vi "SwapInstanceVIUnusedName2 59.vi"(6 "Bindata & descr in":T1, 7 "type":dbl, 8 "error in (no error)":errorcluster, 9 "dims":u8=3 min=1 max=3, 11 "kwarg_name":string="testarg") -> (0 "error out":errorcluster, 1 "Array 3D":dbl[][][](array[numeric]) format="%.2f", 2 "Array 2D":dbl[][](array[numeric]) format="%.2f", 3 "Array 1D":dbl[](array[numeric]) format="%.2f", 4 "Bindata & descr out":T1, 5 "bindata":u8[](array[numeric]))   [LabVIEW 2018]
uses:
  Bindata&description.ctl
  Bindata description.ctl
  bd6e6838-feb3-450b-96c3-bd7f3c631cc0.vi
  c6590a7f-93ce-4676-a9a0-c02eb749ea57.vi
  2ac210e2-aaf9-4bd7-a45e-3c20e6b86e14.vi
  031c4b19-b0b4-4976-a006-513195ae331f.vi
  c6590a7f-93ce-4676-a9a0-c02eb749ea57.vi/81d0cee2-99a7-4483-80a4-f543021384a2.vi
  2ac210e2-aaf9-4bd7-a45e-3c20e6b86e14.vi/3e6cde74-74c6-4a84-975f-0badd6472140.vi
  031c4b19-b0b4-4976-a006-513195ae331f.vi/10b3e457-c1b7-418a-95f2-1100ecc8746c.vi
  c6590a7f-93ce-4676-a9a0-c02eb749ea57.vi/81d0cee2-99a7-4483-80a4-f543021384a2.vi/ea25def5-b33f-46c8-9800-af2b1901f06e.vi
  2ac210e2-aaf9-4bd7-a45e-3c20e6b86e14.vi/3e6cde74-74c6-4a84-975f-0badd6472140.vi/823fcfe4-69d6-4cbf-9d8a-245ae98e7b4b.vi
  031c4b19-b0b4-4976-a006-513195ae331f.vi/10b3e457-c1b7-418a-95f2-1100ecc8746c.vi/6efc0fc5-4d4d-4c58-9f04-a5d9debc7065.vi
  c6590a7f-93ce-4676-a9a0-c02eb749ea57.vi/81d0cee2-99a7-4483-80a4-f543021384a2.vi/ea25def5-b33f-46c8-9800-af2b1901f06e.vi/f81dd119-ed08-4cbe-a226-a8bb7977346c.vi
  2ac210e2-aaf9-4bd7-a45e-3c20e6b86e14.vi/3e6cde74-74c6-4a84-975f-0badd6472140.vi/823fcfe4-69d6-4cbf-9d8a-245ae98e7b4b.vi/7a113b46-2298-43de-997a-f25a7eda3428.vi
  031c4b19-b0b4-4976-a006-513195ae331f.vi/10b3e457-c1b7-418a-95f2-1100ecc8746c.vi/6efc0fc5-4d4d-4c58-9f04-a5d9debc7065.vi/cf528bb0-7ade-42af-b83d-2163692bdb4a.vi
  check ID validity.vi
  LV-Julia_ZMQ-Roundtrip_lib.lvlib
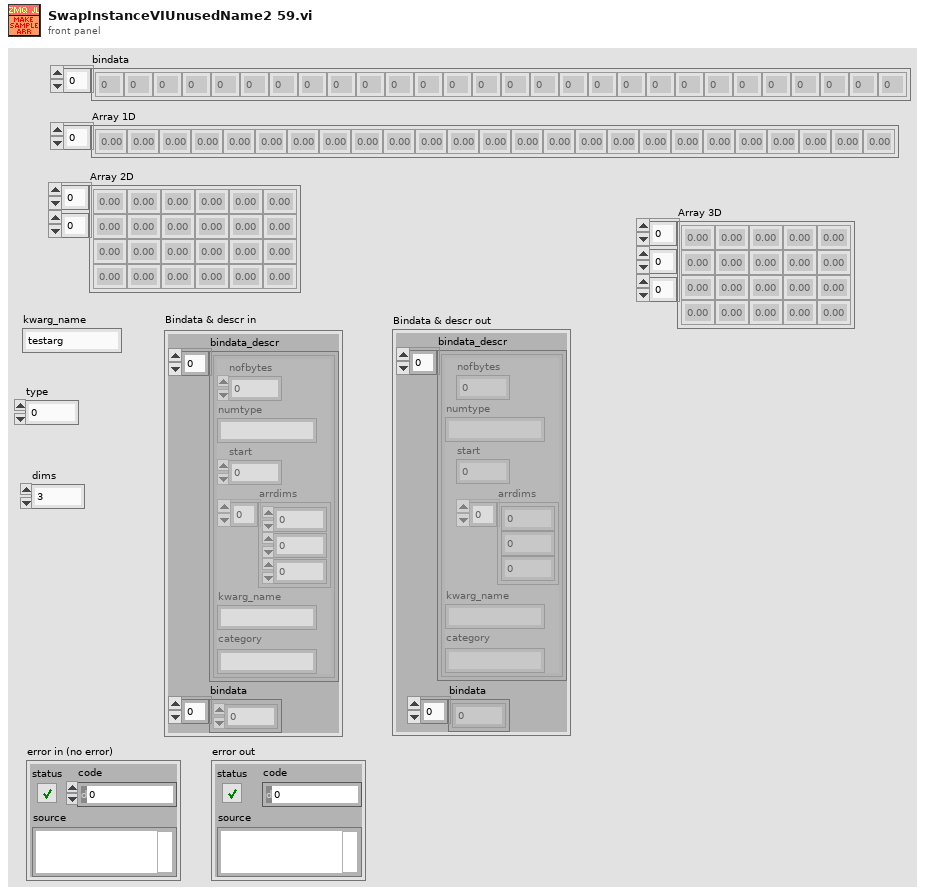
[diagram p1: front panel]
types:
  T1 = typedef "Bindata&description.ctl" = cluster{"bindata_descr":T2[], "bindata":u8[]}
  T2 = typedef "LV-Julia_ZMQ-Roundtrip_lib.lvlib/Bindata description.ctl" = cluster{"nofbytes":i32, "numtype":string, "start":i32, "arrdims":i32[], "kwarg_name":string, "category":string}
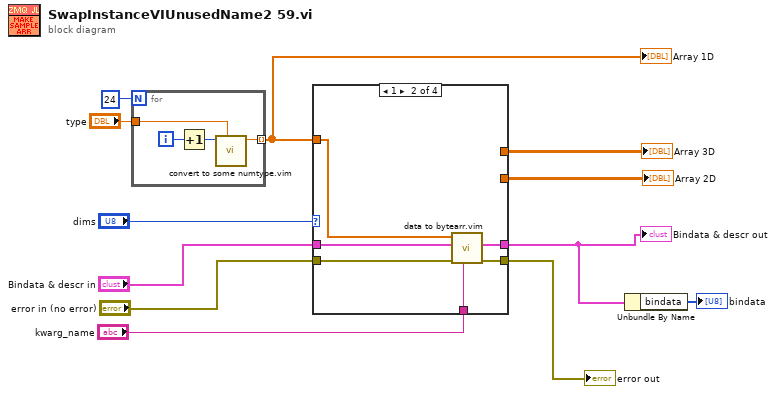
[diagram p0: block diagram]
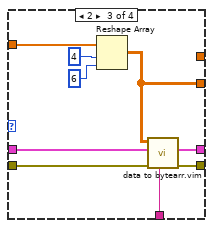
[diagram p3: hidden frame]
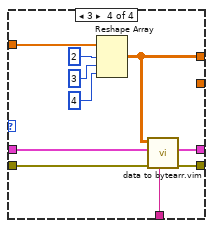
[diagram p4: hidden frame]
diagram:
  n1 = for {
    N: 24 -> [_]
    tunnel: [w14] -> w11 mode=indexing
    tunnel: "type" -> [w13]
    i -> [w16]
    n2 = Increment(x=w16) -> (x+1=w15:i32)
    n3 = call "convert to some numtype.vim"("type"=w13, "Numeric in"=w15) -> ("Numeric out"=w14:dbl)  [unwired: 9 in]
  }
  "Array 1D" <- w11
  n4 = case shown="1" "dims" {
    tunnel: [_ _ _ w42] -> w12
    tunnel: w11 -> [_ w23 w30 w38]
    tunnel: "kwarg_name" -> [_ w22 w29 w37]
    tunnel: "error in (no error)" -> [w17 w21 w28 w36]
    tunnel: [w17 w20 w27 w35] -> w5
    tunnel: [_ w19 w26 w34] -> w2
    tunnel: [_ _ w25 _] -> w4
    tunnel: "Bindata & descr in" -> [_ w18 w24 w33]
    frame 0, Default {
    }
    frame 1 {
      n5 = call "data to bytearr.vim"("kwarg_name"=w22, "error in (no error)"=w21, "Bindata & descr in"=w18, "data in"=w23) -> ("error out"=w20:errorcluster, "Bindata & descr out"=w19:T1)  [unwired: 5 in, 1 out]
    }
    frame 2 {
      n6 = Reshape Array(w30, 4 ("dimension size"), 6 ("dimension size")) -> (w25:dbl[][])
      n7 = call "data to bytearr.vim"("kwarg_name"=w29, "error in (no error)"=w28, "Bindata & descr in"=w24, "data in"=w25) -> ("error out"=w27:errorcluster, "Bindata & descr out"=w26:T1)  [unwired: 5 in, 1 out]
    }
    frame 3 {
      n8 = Reshape Array(w38, 2 ("dimension size"), 3 ("dimension size"), 4 ("dimension size")) -> (w42:dbl[][][])
      n9 = call "data to bytearr.vim"("kwarg_name"=w37, "error in (no error)"=w36, "Bindata & descr in"=w33, "data in"=w42) -> ("error out"=w35:errorcluster, "Bindata & descr out"=w34:T1)  [unwired: 5 in, 1 out]
    }
  }
  "Array 3D" <- w12
  "Bindata & descr out" <- w2
  "error out" <- w5
  "Array 2D" <- w4
  n10 = Unbundle By Name(w2) -> ("bindata"=→"bindata":u8[])
